vi "Chameleon Test Panel.vi"() -> ()   [LabVIEW 2020]
uses:
  <vilib>/Instr/_visa.llb/VISA Configure Serial Port (Instr).vi
panel:
  in  "Quit":bool
  out "Error Out":errorcluster
  in  "VISA Ref":refnum<visa-resource-name>
  in  "Command":string
  out "Response":string
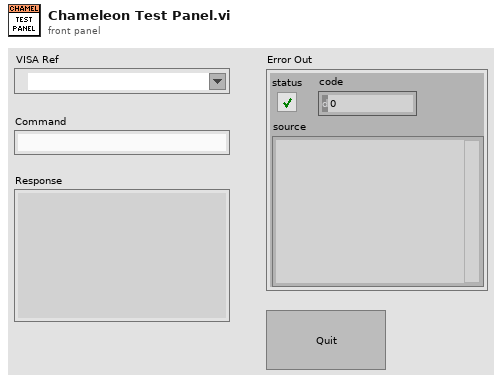
[diagram p1: front panel]
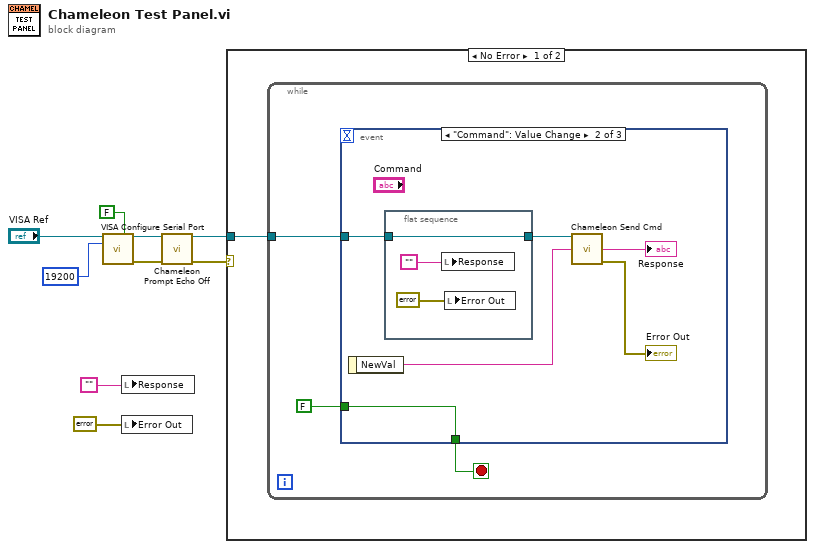
[diagram p0: block diagram]
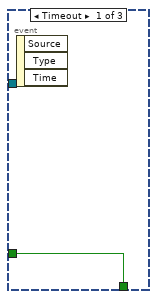
[diagram p2: hidden frame]
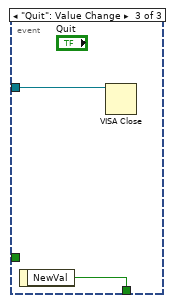
[diagram p3: hidden frame]
diagram:
  n1 = call-poly "VISA Configure Serial Port"("VISA resource name"="VISA Ref", "Enable Termination\nChar (T)"=FALSE ("Enable Termination\nChar (T)"), "baud rate (9600)"=u32 19200) -> ("VISA resource name out"=w4:refnum<visa-resource-name>, "error out"=w3:errorcluster)  [unwired: 11 in]
  n2 = local write "Response"("") -> ()
  n3 = local write "Error Out"(errorcluster {"status"=FALSE, "code"=0, "source"=""} ("error in (no error)")) -> ()
  n4 = call "Chameleon Prompt Echo Off.vi"("VISA Ref"=w4, "Error In"=w3) -> ("VISA Ref Out"=w2:refnum<visa-resource-name>, "Error Out"=w1:errorcluster)  [unwired: 12 in]
  n5 = case shown="No Error" w1 {
    tunnel: w2 -> [w10 _]
    frame No Error {
      n6 = while {
        tunnel: w10 -> [w11]
        stop <- w13 stop-if-true
        n7 = event shown="[1] \"Command\": Value Change" {
          selector: _ -> [_ _ _]
          dyn-events: _ -> [_ _ _]
          timeout: _ -> [_ _ _]
          tunnel: [w14 w20 w25] -> w13
          tunnel: FALSE -> [w14 w20 _]
          tunnel: w11 -> [_ w17 w24]
          event Timeout {
            n8 = event-data() -> ()  [unwired: 1 in, 3 out]
          }
          event "Command": Value Change {
            n9 = event-data() -> ("NewVal"=w15:string)  [unwired: 1 in]
            n10 = flat-sequence {
              tunnel: w17 -> [w23]
              tunnel: [w23] -> w16
              frame #0 {
                n11 = local write "Response"("") -> ()
                n12 = local write "Error Out"(errorcluster {"status"=FALSE, "code"=0, "source"=""} ("error in (no error)")) -> ()
              }
            }
            n13 = call "Chameleon Send Cmd.vi"("VISA Ref"=w16, "Command"=w15) -> ("Response"=→"Response":string, "Error Out"=→"Error Out":errorcluster)  [unwired: 11 in, 1 out]
          }
          event "Quit": Value Change {
            n14 = event-data() -> ("NewVal"=w25:bool)  [unwired: 1 in]
            n15 = VISA Close(VISA resource name=w24) -> ()  [unwired: 1 in, 1 out]
          }
        }
      }
    }
    frame Error {
    }
  }
